vi "nipkg-createPackageTemplate.vi"() -> ()   [LabVIEW 2014, in "nipkg-build-system.lvlib"]
uses:
  nipkg-build-system.lvlib
  <vilib>/Wiresmith Technology/LabVIEW CLI/CLI Class/CLI.lvclass
panel:
  out "error out":errorcluster
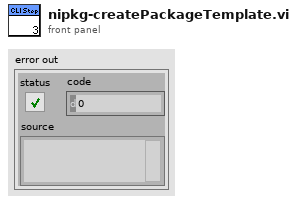
[diagram p1: front panel]
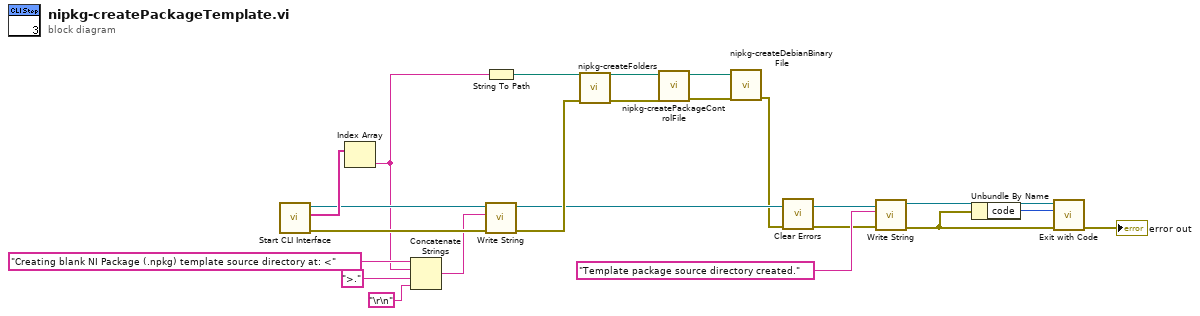
[diagram p0: block diagram]
diagram:
  n1 = call <vilib>:"Start CLI Interface.vi"() -> ("error out"=w14:errorcluster, "Custom Parameters"=w19:string[], "CLI out"=w15:refnum<class "CLI.lvclass">)  [unwired: 9 in]
  n2 = Index Array(array=w19) -> (element=w10:string)  [unwired: 1 in]
  n3 = Concatenate Strings("Creating blank NI Package (.npkg) template source directory at: <" ("string"), w10, ">." ("string"), "\r\n") -> (w13:string)
  n4 = String To Path(string=w10) -> (path=w9:path)
  n5 = call <vilib>:"Write String.vi"("error in (no error)"=w14, "Text to Write"=w13, "CLI in"=w15) -> ("error out"=w12:errorcluster, "CLI out"=w8:refnum<class "CLI.lvclass">)  [unwired: 7 in]
  n6 = call "nipkg-createFolders.vi"("error in (no error)"=w12, "New package source directory"=w9) -> ("error out"=w11:errorcluster, "Package source directory out"=w22:path)  [unwired: 8 in]
  n7 = call "nipkg-createPackageControlFile.vi"("error in (no error)"=w11, "Package directory"=w22) -> ("error out"=w21:errorcluster, "Package directory out"=w20:path)  [unwired: 8 in]
  n8 = call "nipkg-createDebianBinaryFile.vi"("error in (no error)"=w21, "Package directory"=w20) -> ("error out"=w2:errorcluster)  [unwired: 8 in, 1 out]
  n9 = call <vilib>:"Clear Errors.vi"("error in (no error)"=w2) -> ("error out"=w1:errorcluster)  [unwired: 5 in, 1 out]
  n10 = call <vilib>:"Write String.vi"("error in (no error)"=w1, "Text to Write"="Template package source directory created.", "CLI in"=w8) -> ("error out"=w6:errorcluster, "CLI out"=w7:refnum<class "CLI.lvclass">)  [unwired: 7 in]
  n11 = Unbundle By Name(w6) -> ("code"=w5:i32)
  n12 = call <vilib>:"Exit with Code.vi"("error in (no error)"=w6, "Exit Code (0)"=w5, "CLI in"=w7) -> ("error out"=→"error out":errorcluster)  [unwired: 8 in]
